vi "Endurance.vi"() -> ()   [LabVIEW 2020]
uses:
  Control/EnduranceIndicator.ctl
  Control/EnduranceBufferControl.ctl
  Control/EnduranceRecordRemove.ctl
  Control/EnduranceCurrentIndicator.ctl
  Control/EnduranceState.ctl
  <vilib>/DAQmx/write.llb/DAQmx Write (Analog DBL 1Chan 1Samp).vi
  <vilib>/DAQmx/read.llb/DAQmx Read (Analog DBL 1Chan 1Samp).vi
  <vilib>/DAQmx/create/channels.llb/DAQmx Create Channel (AO-Voltage-Basic).vi
  <vilib>/DAQmx/create/channels.llb/DAQmx Create Channel (AI-Voltage-Basic).vi
  <vilib>/Utility/file.llb/Read Delimited Spreadsheet (string).vi
  <vilib>/DAQmx/miscellaneous.llb/DAQmx Fill In Error Info.vi
panel:
  out "CurrentIndicator":T1
  out "ElapsedTime":string
  in  "RecordRemove":T2
  in  "BufferControl":T3
  in  "DeviceName":tag
  out "BufferIndicator":T4
  in  "Ready":bool
  in  "Stop":bool
  # "2022 KSAE Formula Endurance  Event"
  # "Record-6:"
  # "Record-7:"
  # "Record-8:"
  # "Record-9:"
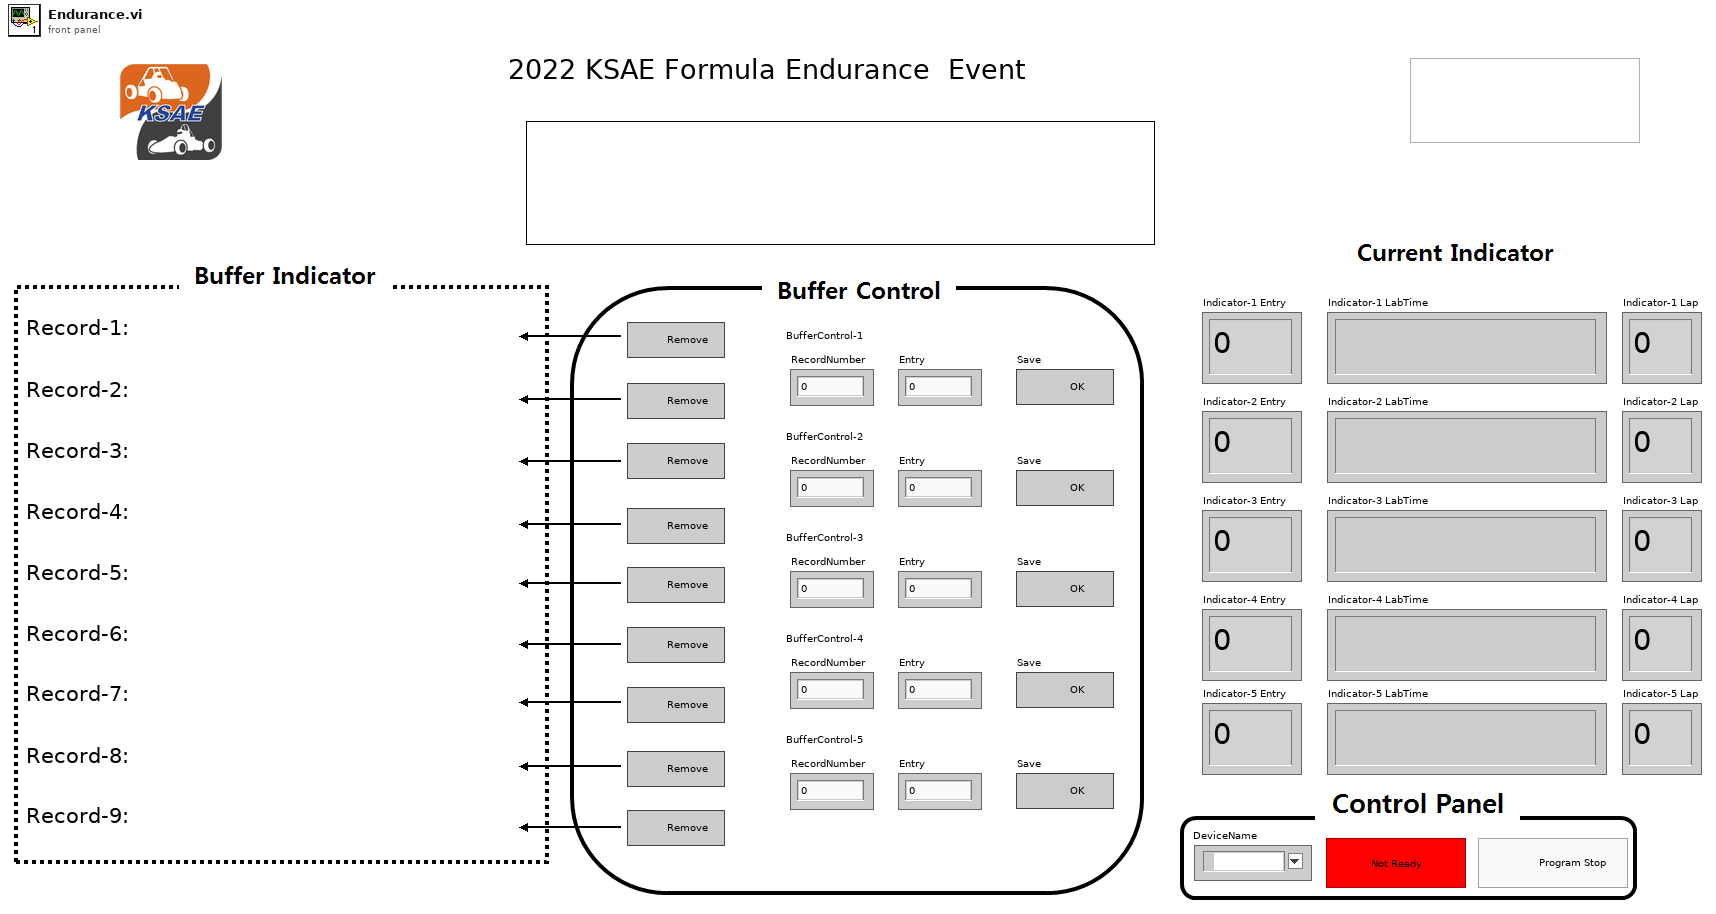
[diagram p1: front panel]
types:
  T1 = typedef "EnduranceCurrentIndicator.ctl" = cluster{"Indicator-1 Entry":u8, "Indicator-1 LabTime":string, "Indicator-1 Lap":u8, "Indicator-2 Entry":u8, "Indicator-2 LabTime":string, "Indicator-2 Lap":u8, "Indicator-3 Entry":u8, "Indicator-3 LabTime":string, "Indicator-3 Lap":u8, "Indicator-4 Entry":u8, "Indicator-4 LabTime":string, "Indicator-4 Lap":u8, "Indicator-5 Entry":u8, "Indicator-5 LabTime":string, "Indicator-5 Lap":u8}
  T2 = typedef "EnduranceRecordRemove.ctl" = cluster{"Record-1 Remove":bool, "Record-2 Remove":bool, "Record-3 Remove":bool, "Record-4 Remove":bool, "Record-5 Remove":bool, "Record-6 Remove":bool, "Record-7 Remove":bool, "Record-8 Remove":bool, "Record-9 Remove":bool}
  T3 = typedef "EnduranceBufferControl.ctl" = cluster{"BufferControl-1":cluster{"RecordNumber":u8, "Entry":u8, "Save":bool}, "BufferControl-2":cluster{"RecordNumber":u8, "Entry":u8, "Save":bool}, "BufferControl-3":cluster{"RecordNumber":u8, "Entry":u8, "Save":bool}, "BufferControl-4":cluster{"RecordNumber":u8, "Entry":u8, "Save ":bool}, "BufferControl-5":cluster{"RecordNumber":u8, "Entry":u8, "Save":bool}}
  T4 = typedef "EnduranceIndicator.ctl" = cluster{"Record-1":string, "Record-2":string, "Record-3":string, "Record-4":string, "Record-5":string, "Record-6":string, "Record-7":string, "Record-8":string, "Record-9":string}
  T5 = typedef "EnduranceState.ctl" = enum16{"Initial", "Ready", "Running", "LoggingData", "ProgramStop"}
  T6 = cluster{"BufferIndicator":T4, "State":T5, "InitialTime":i64, "RecordBuffer":cluster{"RecordBuffer(Time)":i64[], "RecordBuffer(Display)":string[]}, "CurrentIndicator":T1, "BufferControl":T3}
  T7 = cluster{"RecordBuffer(Time)":i64[], "RecordBuffer(Display)":string[]}
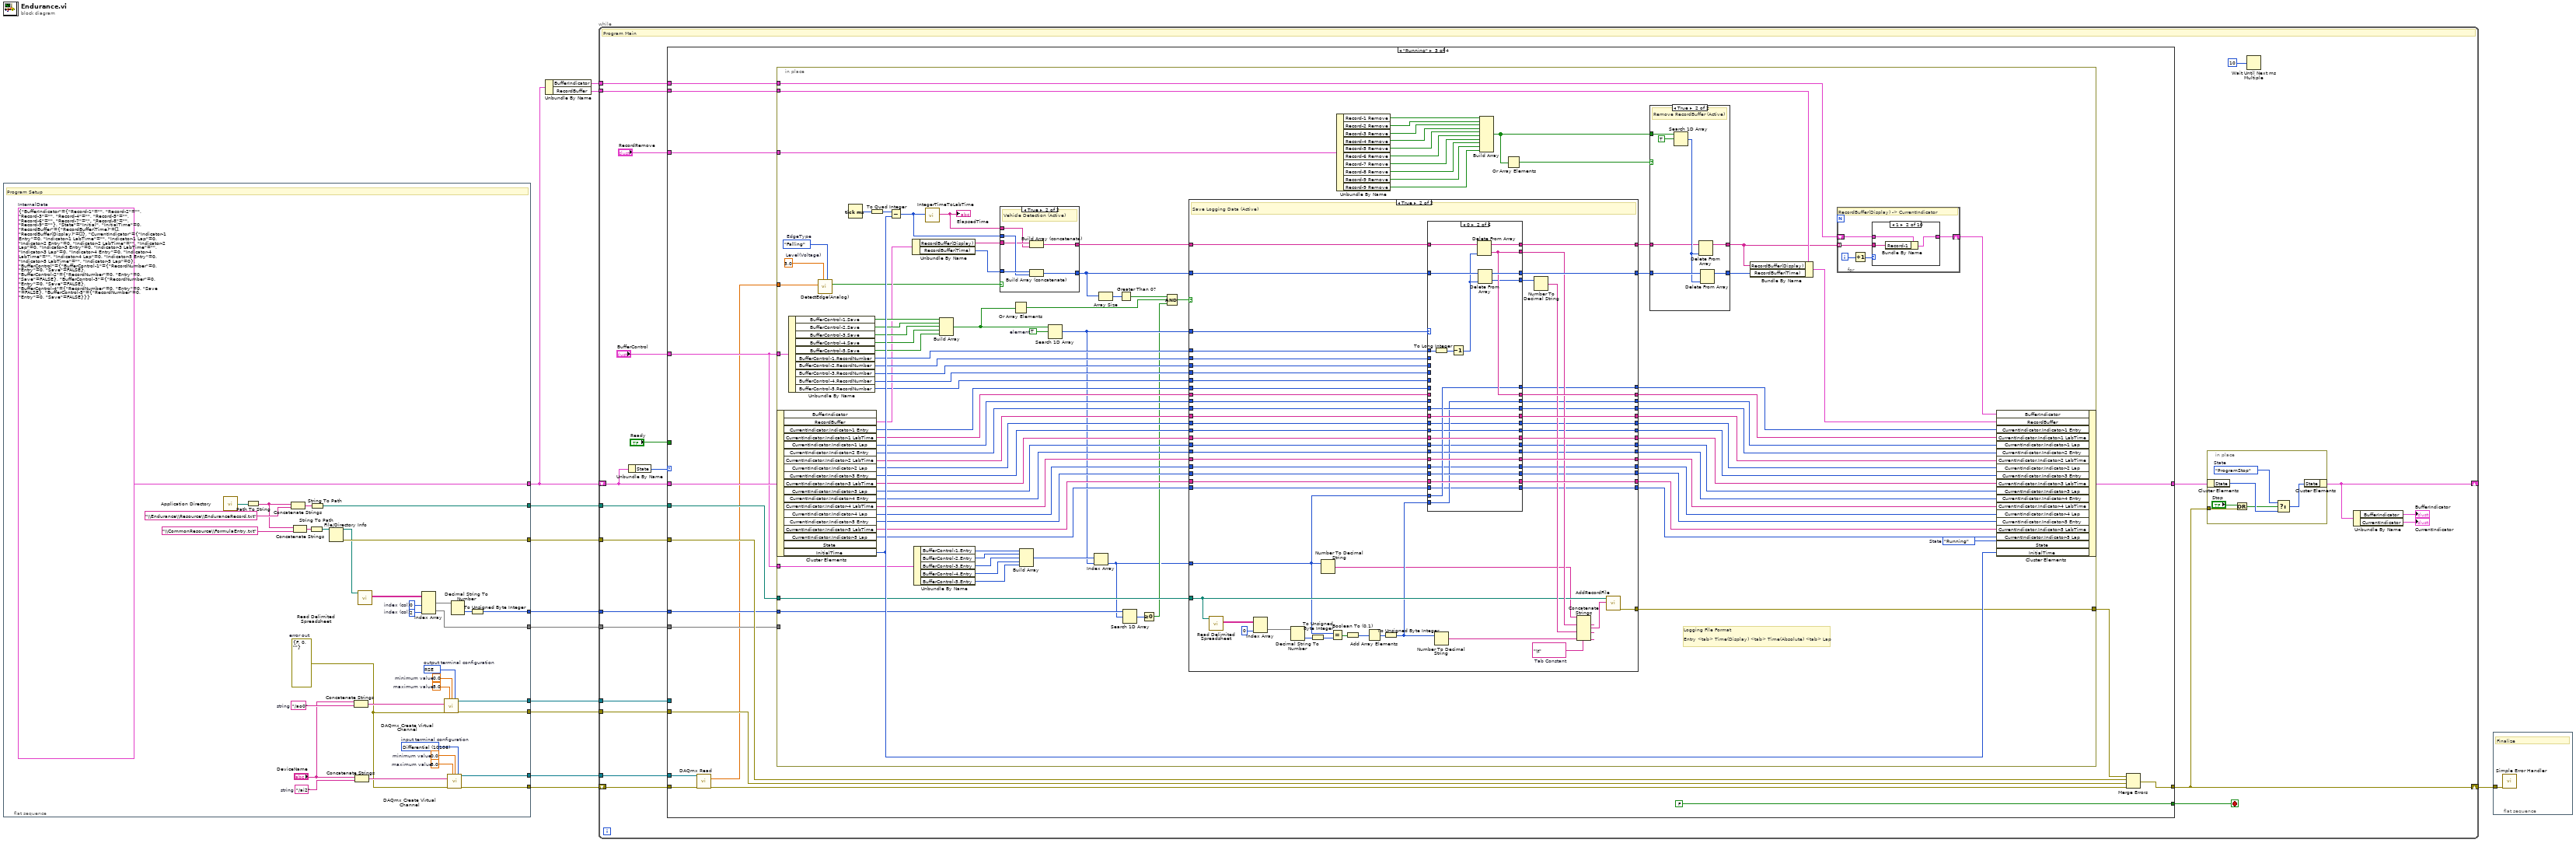
[diagram p0: block diagram]
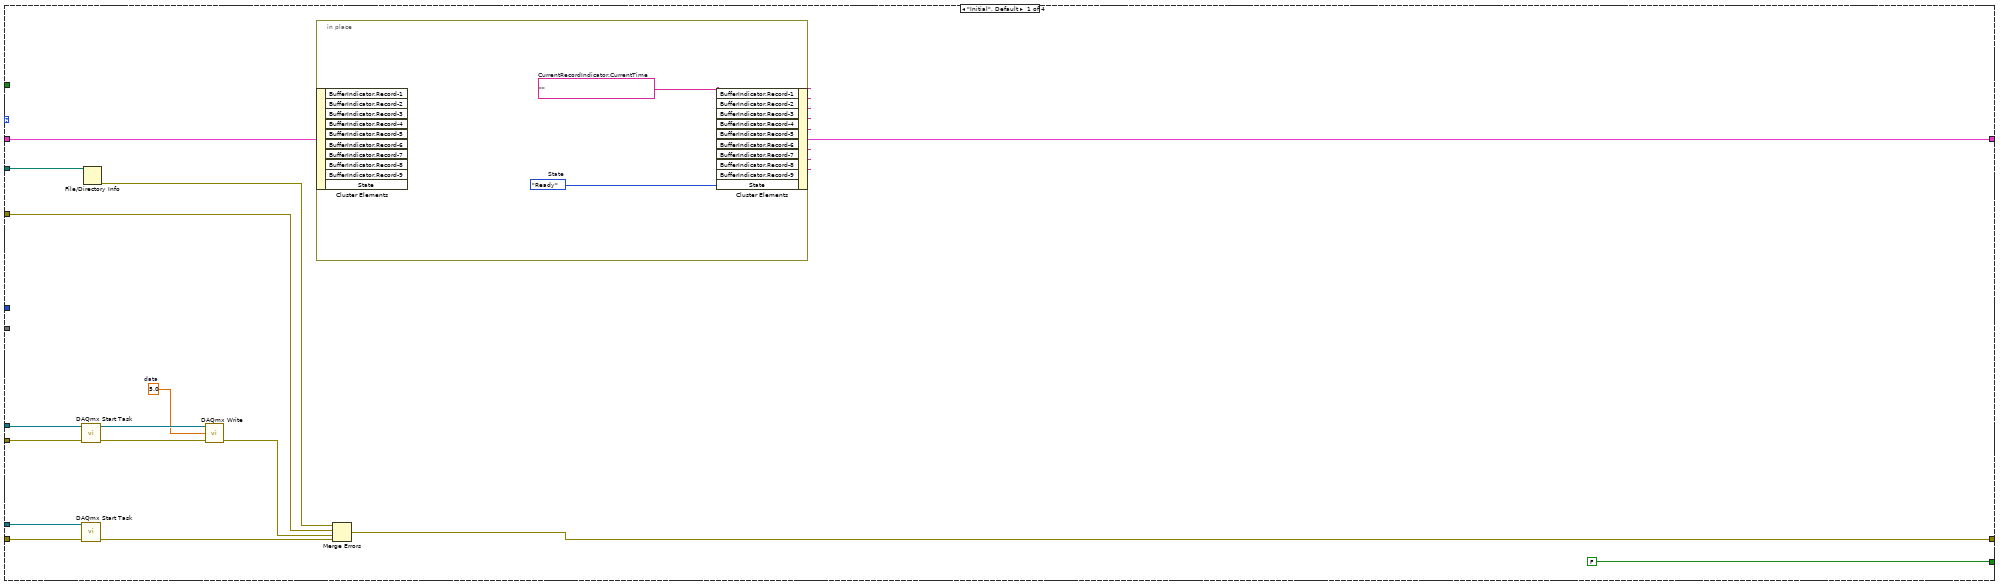
[diagram p2: hidden frame]
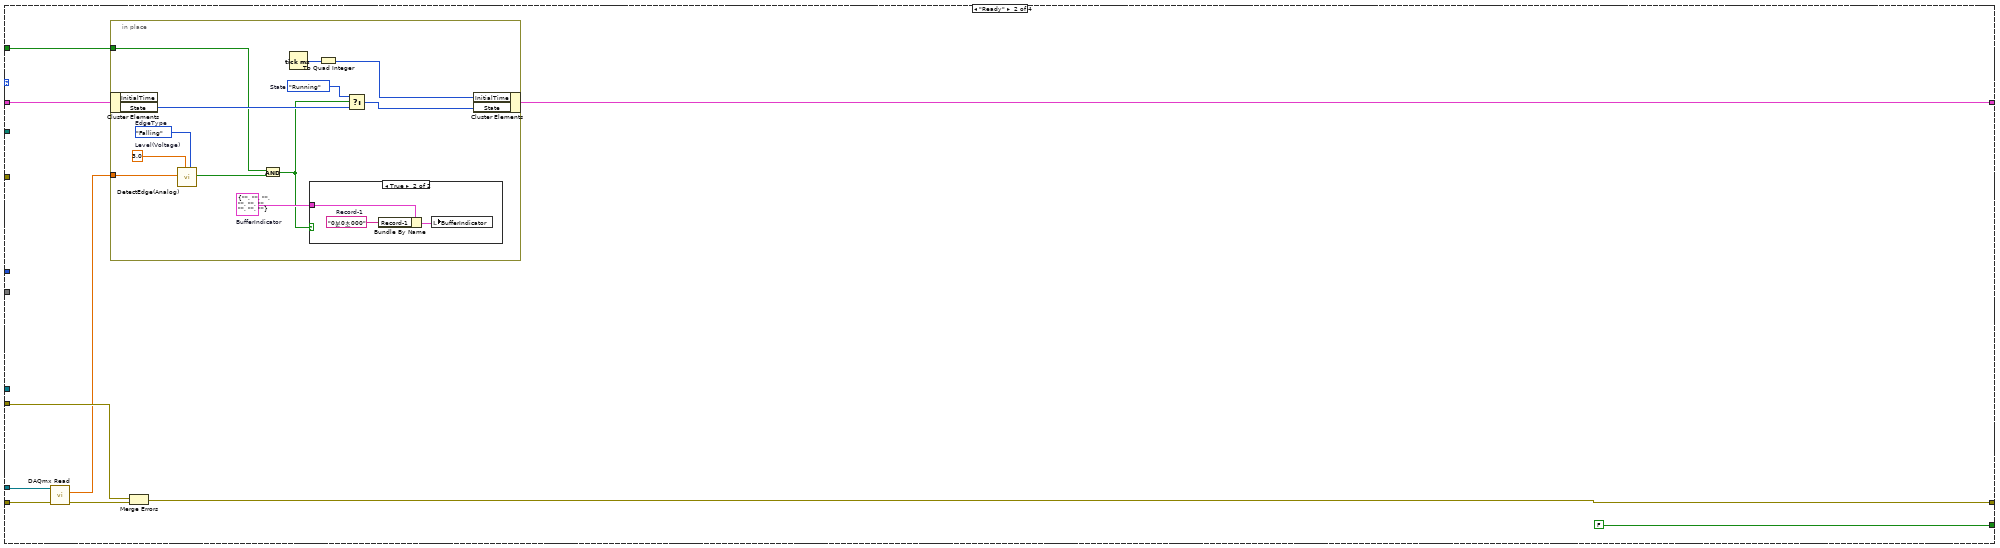
[diagram p3: hidden frame]
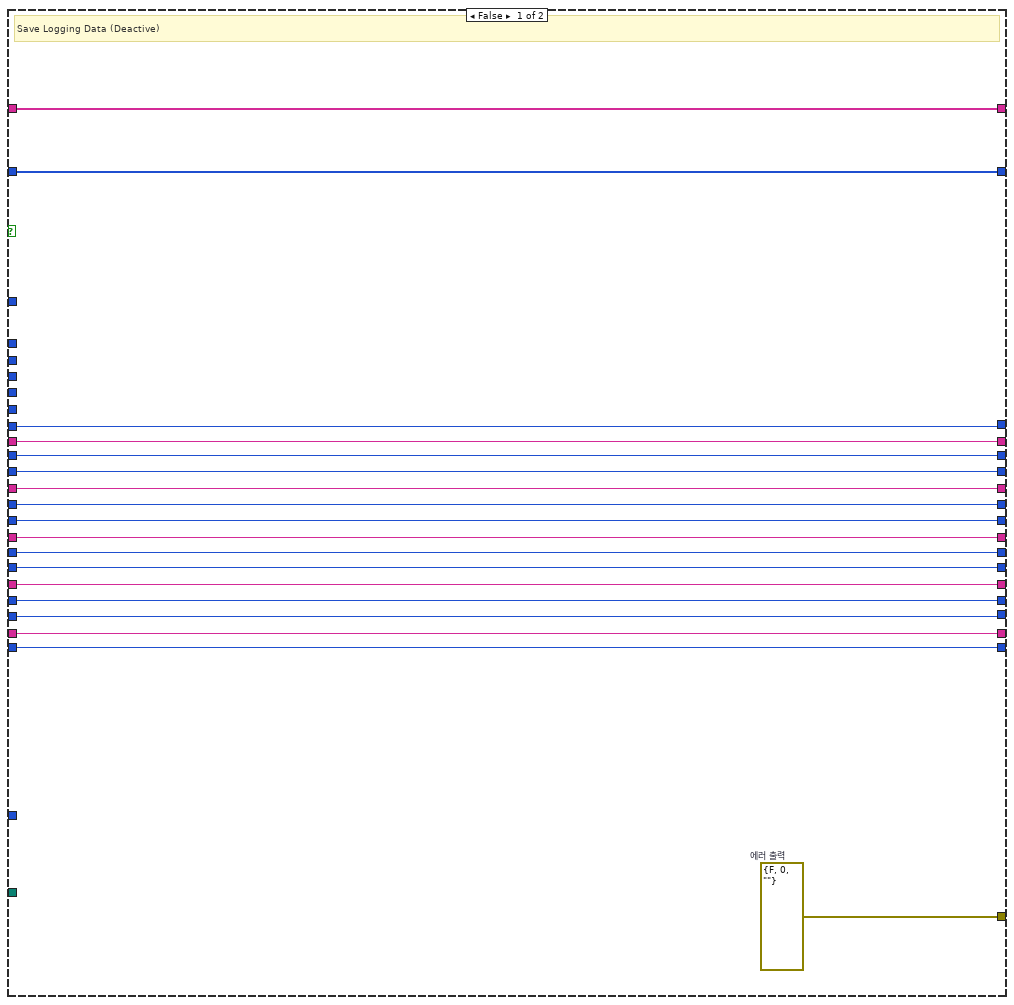
[diagram p6: hidden frame]
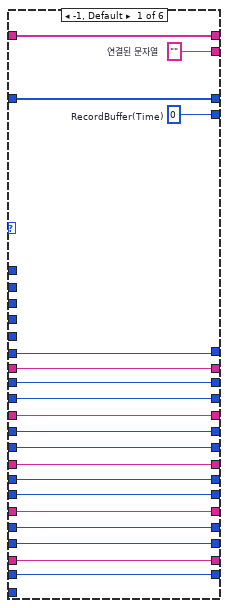
[diagram p7: hidden frame]
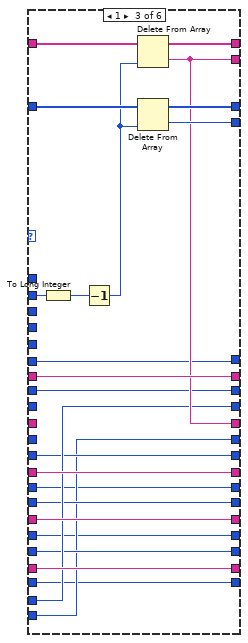
[diagram p8: hidden frame]
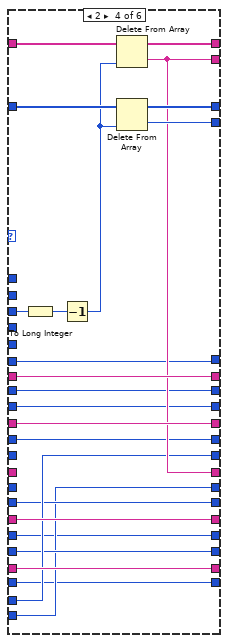
[diagram p9: hidden frame]
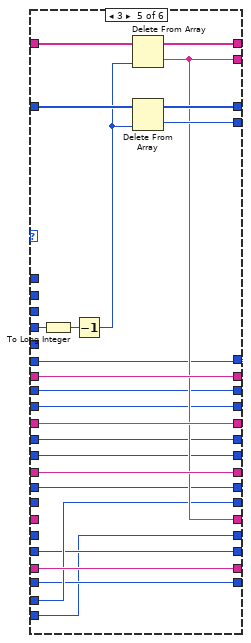
[diagram p10: hidden frame]
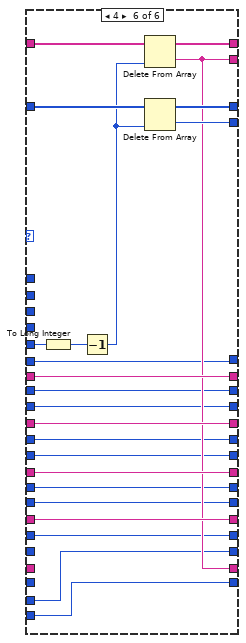
[diagram p11: hidden frame]
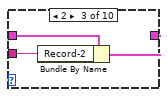
[diagram p14: hidden frame]
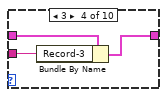
[diagram p15: hidden frame]
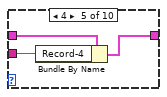
[diagram p16: hidden frame]
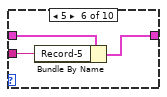
[diagram p17: hidden frame]
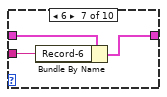
[diagram p18: hidden frame]
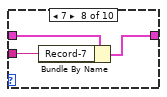
[diagram p19: hidden frame]
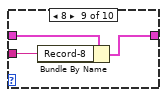
[diagram p20: hidden frame]
diagram:
  n1 = flat-sequence {
    tunnel: [w45] -> w11
    tunnel: [w44] -> w10
    tunnel: [w41] -> w9
    tunnel: [w40] -> w8
    tunnel: [w36] -> w6
    tunnel: [w27] -> w7
    tunnel: [w22] -> w3
    tunnel: [w15] -> w2
    tunnel: [w17] -> w1
    frame #0 {
      w13 = errorcluster {"status"=FALSE, "code"=0, "source"=""}  # error out
      w19 = 2  # index (col)
      w20 = 0  # index (col)
      w36 = T6 {"BufferIndicator"={"Record-1"="", "Record-2"="", "Record-3"="", "Record-4"="", "Record-5"="", "Record-6"="", "Record-7"="", "Record-8"="", "Record-9"=""}, "State"=enum."Initial", "InitialTime"=0, "RecordBuffer"={"RecordBuffer(Time)"=[], "RecordBuffer(Display)"=[]}, "CurrentIndicator"={"Indicator-1 Entry"=0, "Indicator-1 LabTime"="", "Indicator-1 Lap"=0, "Indicator-2 Entry"=0, "Indicator-2 LabTime"="", "Indicator-2 Lap"=0, "Indicator-3 Entry"=0, "Indicator-3 LabTime"="", "Indicator-3 Lap"=0, "Indicator-4 Entry"=0, "Indicator-4 LabTime"="", "Indicator-4 Lap"=0, "Indicator-5 Entry"=0, "Indicator-5 LabTime"="", "Indicator-5 Lap"=0}, "BufferControl"={"BufferControl-1"={"RecordNumber"=0, "Entry"=0, "Save"=FALSE}, "BufferControl-2"={"RecordNumber"=0, "Entry"=0, "Save"=FALSE}, "BufferControl-3"={"RecordNumber"=0, "Entry"=0, "Save"=FALSE}, "BufferControl-4"={"RecordNumber"=0, "Entry"=0, "Save "=FALSE}, "BufferControl-5"={"RecordNumber"=0, "Entry"=0, "Save"=FALSE}}}  # InternalData
      w33 = "/ai2"  # string
      w35 = "/ao0"  # string
      w37 = 10083 items=["Default"=-1, "RSE"=10083, "Differential"=10106, "Pseudodifferential"=12529]  # output terminal configuration
      w38 = 0.0  # minimum value
      w39 = 5.0  # maximum value
      w43 = 5.0  # maximum value
      w42 = 0.0  # minimum value
      w46 = 10106 items=["default"=-1, "RSE"=10083, "NRSE"=10078, "Differential"=10106, "Pseudodifferential"=12529]  # input terminal configuration
      # "Program Setup"
      n2 = call <vilib>:"Application Directory.vi"() -> ("Application Directory"=w30:path)
      n3 = Path To String(path=w30) -> (string=w24:string)
      n4 = Concatenate Strings "Concatenate Strings"(w24, "\\Endurance\\Resource\\EnduranceRecord.txt") -> (w28:string)
      n5 = Concatenate Strings "Concatenate Strings"(w24, "\\CommonResource\\FormulaEntry.txt") -> (w25:string)
      n6 = String To Path(string=w25) -> (path=w23:path)
      n7 = String To Path(string=w28) -> (path=w27:path)
      n8 = File/Directory Info(path=w23) -> (path out=w21:path, error out=w22:errorcluster)  [unwired: 1 in, 5 out]
      n9 = Concatenate Strings "Concatenate Strings"("DeviceName", w35) -> (w32:string)
      n10 = Concatenate Strings "Concatenate Strings"("DeviceName", w33) -> (w31:string)
      n11 = call-poly <vilib>:"Read Delimited Spreadsheet.vi"("file path (dialog if empty)"=w21) -> ("all rows"=w14:string[][])  [unwired: 9 in, 5 out]
      n12 = Index Array "Index Array"(array=w14, index (col) #1=w20, index (col) #2=w19) -> (element #1=w18:string[], element #2=w17:string[])  [unwired: 2 in]
      n13 = call-poly <vilib>:"DAQmx Create Virtual Channel.vi"("maximum value"=w39, "minimum value"=w38, "output terminal configuration"=w37, "physical channels"=w32, "error in"=w13) -> ("task out"=w41:refnum<k21>, "error out"=w40:errorcluster)  [unwired: 9 in]
      n14 = call-poly <vilib>:"DAQmx Create Virtual Channel.vi"("maximum value"=w43, "minimum value"=w42, "input terminal configuration"=w46, "physical channels"=w31, "error in"=w13) -> ("task out"=w44:refnum<k21>, "error out"=w45:errorcluster)  [unwired: 9 in]
      n15 = Decimal String To Number(string=w18) -> (number=w16:i32[])  [unwired: 2 in, 1 out]
      n16 = To Unsigned Byte Integer(number=w16) -> (unsigned 8bit integer=w15:u8[])
    }
  }
  n17 = Unbundle By Name(w6) -> ("BufferIndicator"=w4:T4, "RecordBuffer"=w5:T7)
  n18 = while {
    tunnel: w10 -> [w68]
    shift-right: [w58] -> _
    shift-left: w6 -> [w65]
    shift-right: [w62] -> w12
    shift-left: w11 -> [w67]
    tunnel: w9 -> [w60]
    tunnel: w8 -> [w59]
    tunnel: w7 -> [w54]
    tunnel: w5 -> [w53]
    tunnel: w4 -> [w52]
    tunnel: w3 -> [w50]
    tunnel: w2 -> [w49]
    tunnel: w1 -> [w48]
    stop <- w63 stop-if-true
    # "Program Main"
    n19 = Unbundle By Name(w65) -> ("State"=w66:T5)
    n20 = case shown="\"Running\"" w66 {
      tunnel: w68 -> [w77 w96 w129 w495]
      tunnel: w67 -> [w78 w95 w128 w498]
      tunnel: w65 -> [w84 w94 w125 w497]
      tunnel: [w83 w93 w126 w496] -> w64
      tunnel: [FALSE FALSE FALSE TRUE] -> w63
      tunnel: [w81 w89 w124 w490] -> w62
      tunnel: "Ready" -> [_ w90 _ _]
      tunnel: w60 -> [w74 _ _ w492]
      tunnel: w59 -> [w75 w88 w123 w491]
      tunnel: "BufferControl" -> [_ _ w118 _]
      tunnel: "RecordRemove" -> [_ _ w121 _]
      tunnel: w54 -> [w70 _ w120 _]
      tunnel: w53 -> [_ _ w117 _]
      tunnel: w52 -> [_ _ w116 _]
      tunnel: w50 -> [w69 _ w115 w488]
      tunnel: w49 -> [_ _ w114 _]
      tunnel: w48 -> [_ _ w113 _]
      frame "Initial", Default {
        w72 = 5.0  # data
        n21 = call <vilib>:"DAQmx Start Task.vi"("task/channels in"=w74, "error in"=w75) -> ("task out"=w80:refnum<k21>, "error out"=w79:errorcluster)  [unwired: 12 in]
        n22 = call <vilib>:"DAQmx Start Task.vi"("task/channels in"=w77, "error in"=w78) -> ("error out"=w76:errorcluster)  [unwired: 12 in, 1 out]
        n23 = File/Directory Info(path=w70) -> (error out=w71:errorcluster)  [unwired: 1 in, 6 out]
        n24 = call-poly <vilib>:"DAQmx Write.vi"("task/channels in"=w80, "data"=w72, "error in"=w79) -> ("error out"=w73:errorcluster)  [unwired: 10 in, 2 out]
        n25 = in-place {
          w85 = EnduranceState."Ready"  # State
          w86 = ""  # CurrentRecordIndicator.CurrentTime
          n26 = in-place-cluster #1(w84) -> ()  [unwired: 10 out]
          n27 = in-place-cluster #1("BufferIndicator.Record-1"=w86, "BufferIndicator.Record-2"=w86, "BufferIndicator.Record-3"=w86, "BufferIndicator.Record-4"=w86, "BufferIndicator.Record-5"=w86, "BufferIndicator.Record-6"=w86, "BufferIndicator.Record-7"=w86, "BufferIndicator.Record-8"=w86, "BufferIndicator.Record-9"=w86, "State"=w85) -> (w83:T6)
        }
        n28 = Merge Errors "Merge Errors"(w71, w69, w73, w76) -> (w81:errorcluster)
      }
      frame "Ready" {
        n29 = call-poly <vilib>:"DAQmx Read.vi"("task/channels in"=w96, "error in"=w95) -> ("data"=w87:dbl, "error out"=w91:errorcluster)  [unwired: 11 in, 1 out]
        n30 = in-place {
          in-place-border: w87 -> [w105]
          in-place-border: w90 -> [w103]
          w98 = enum16{"Rising", "Falling"}."Falling"  # EdgeType
          w100 = T4 {"Record-1"="", "Record-2"="", "Record-3"="", "Record-4"="", "Record-5"="", "Record-6"="", "Record-7"="", "Record-8"="", "Record-9"=""}  # BufferIndicator
          w102 = EnduranceState."Running"  # State
          w104 = 3.0  # Level(Voltage)
          n31 = in-place-cluster #2(w94) -> ("State"=w108:T5)  [unwired: 1 out]
          n32 = call "DetectEdge(Analog).vi"("EdgeType"=w98, "Level(Voltage)"=w104, "Voltage"=w105) -> ("DetectedEdge"=w106:bool)  [unwired: 8 in]
          n33 = And(x=w103, y=w106) -> (x .and. y?=w99:bool)
          n34 = Tick Count (ms)() -> (millisecond timer value=w101:u32)
          n35 = case shown="True" w99 {
            tunnel: w100 -> [_ w111]
            frame False {
            }
            frame True {
              w109 = "0분0초000"  # Record-1
              n36 = Bundle By Name(cluster=w111, "Record-1"=w109) -> (w110:T4)
              n37 = local write "BufferIndicator"(w110) -> ()
            }
          }
          n38 = To Quad Integer(1:w101) -> (0:w97:i64)
          n39 = Select(t=w102, s=w99, f=w108) -> (s? t:f=w107:T5)
          n40 = in-place-cluster #2("InitialTime"=w97, "State"=w107) -> (w93:T6)
        }
        n41 = Merge Errors "Merge Errors"(w88, w91) -> (w89:errorcluster)
      }
      frame "Running" {
        n42 = call-poly <vilib>:"DAQmx Read.vi"("task/channels in"=w129, "error in"=w128) -> ("data"=w112:dbl, "error out"=w122:errorcluster)  [unwired: 11 in, 1 out]
        n43 = in-place {
          in-place-border: w112 -> [w224]
          in-place-border: w118 -> [w183]
          in-place-border: w121 -> [w214]
          in-place-border: w120 -> [w185]
          in-place-border: [w184] -> w119
          in-place-border: w118 -> [w182]
          in-place-border: w117 -> [w172]
          in-place-border: w116 -> [w170]
          in-place-border: w114 -> [w135]
          in-place-border: w113 -> [_]
          w130 = enum16{"Rising", "Falling"}."Falling"  # EdgeType
          w144 = TRUE  # element
          w169 = EnduranceState."Running"  # State
          w226 = 3.0  # Level(Voltage)
          # "Logging File Format\n\nEntry <tab> Time(Display) <tab> Time(Absolute) <tab> Lap"
          n44 = in-place-cluster #3(w125) -> ("RecordBuffer"=w178:T7, "CurrentIndicator.Indicator-1 Entry"=w167:u8, "CurrentIndicator.Indicator-1 LabTime"=w195:string, "CurrentIndicator.Indicator-1 Lap"=w154:u8, "CurrentIndicator.Indicator-2 Entry"=w165:u8, "CurrentIndicator.Indicator-2 LabTime"=w194:string, "CurrentIndicator.Indicator-2 Lap"=w152:u8, "CurrentIndicator.Indicator-3 Entry"=w163:u8, "CurrentIndicator.Indicator-3 LabTime"=w193:string, "CurrentIndicator.Indicator-3 Lap"=w150:u8, "CurrentIndicator.Indicator-4 Entry"=w161:u8, "CurrentIndicator.Indicator-4 LabTime"=w192:string, "CurrentIndicator.Indicator-4 Lap"=w148:u8, "CurrentIndicator.Indicator-5 Entry"=w159:u8, "CurrentIndicator.Indicator-5 LabTime"=w191:string, "CurrentIndicator.Indicator-5 Lap"=w146:u8, "InitialTime"=w225:i64)  [unwired: 2 out]
          n45 = Unbundle By Name(w183) -> ("BufferControl-1.Save"=w201:bool, "BufferControl-2.Save"=w200:bool, "BufferControl-3.Save"=w199:bool, "BufferControl-4.Save"=w198:bool, "BufferControl-5.Save"=w197:bool, "BufferControl-1.RecordNumber"=w218:u8, "BufferControl-2.RecordNumber"=w217:u8, "BufferControl-3.RecordNumber"=w216:u8, "BufferControl-4.RecordNumber"=w215:u8, "BufferControl-5.RecordNumber"=w168:u8)
          n46 = call "DetectEdge(Analog).vi"("EdgeType"=w130, "Level(Voltage)"=w226, "Voltage"=w224) -> ("DetectedEdge"=w131:bool)  [unwired: 8 in]
          n47 = Tick Count (ms)() -> (millisecond timer value=w223:u32)
          n48 = To Quad Integer(1:w223) -> (0:w222:i64)
          n49 = Subtract(x=w222, y=w225) -> (x-y=w221:i64)
          n50 = Unbundle By Name(w178) -> ("RecordBuffer(Display)"=w176:string[], "RecordBuffer(Time)"=w177:i64[])
          n51 = Unbundle By Name(w182) -> ("BufferControl-1.Entry"=w142:u8, "BufferControl-2.Entry"=w141:u8, "BufferControl-3.Entry"=w140:u8, "BufferControl-4.Entry"=w139:u8, "BufferControl-5.Entry"=w138:u8)
          n52 = call "IntegerTimeToLabTime.vi"("inputTime(msec)"=w221) -> ("outputTime(mm-ss-sss)"=w175:string)  [unwired: 10 in]
          "ElapsedTime" <- w175
          n53 = Build Array "Build Array"(w201, w200, w199, w198, w197) -> (w143:bool[])
          n54 = case shown="True" w131 {
            tunnel: w177 -> [w228 w234]
            tunnel: w221 -> [_ w232]
            tunnel: [w228 w233] -> w181
            tunnel: w176 -> [w227 w231]
            tunnel: w175 -> [_ w230]
            tunnel: [w227 w229] -> w174
            frame False {
              # "Vehicle Detection (Deactive)"
            }
            frame True {
              # "Vehicle Detection (Active)"
              n55 = Build Array (concatenate) "Build Array"(w231, w230) -> (w229:string[])
              n56 = Build Array (concatenate) "Build Array"(w234, w232) -> (w233:i64[])
            }
          }
          n57 = Or Array Elements(Boolean array=w143) -> (logical OR=w180:bool)
          n58 = Build Array "Build Array"(w142, w141, w140, w139, w138) -> (w137:u8[])
          n59 = Search 1D Array(1D array=w143, element=w144) -> (index of element=w136:i32)  [unwired: 1 in]
          n60 = Index Array "Index Array"(array=w137, index=w136) -> (element=w133:u8)
          n61 = Array Size(array=w181) -> (size(s)=w220:i32)
          n62 = Greater Than 0?(x=w220) -> (x > 0?=w196:bool)
          n63 = Search 1D Array(1D array=w135, element=w133) -> (index of element=w132:i32)  [unwired: 1 in]
          n64 = Greater Or Equal To 0?(x=w132) -> (x >= 0?=w134:bool)
          n65 = Compound Arithmetic op=AND(w196, w180, w134) -> (w219:bool)
          n66 = case shown="True" w219 {
            tunnel: w181 -> [w246 w311]
            tunnel: [w246 w294] -> w179
            tunnel: w218 -> [_ w310]
            tunnel: w217 -> [_ w309]
            tunnel: w216 -> [_ w308]
            tunnel: w215 -> [_ w307]
            tunnel: w168 -> [_ w306]
            tunnel: w195 -> [w252 w305]
            tunnel: w194 -> [w251 w304]
            tunnel: w193 -> [w250 w303]
            tunnel: w192 -> [w249 w302]
            tunnel: w191 -> [w248 w301]
            tunnel: [w252 w300] -> w190
            tunnel: [w251 w299] -> w189
            tunnel: [w250 w298] -> w188
            tunnel: [w249 w297] -> w187
            tunnel: [w248 w296] -> w186
            tunnel: w185 -> [_ w278]
            tunnel: [w247 w295] -> w184
            tunnel: [w245 w292] -> w173
            tunnel: w174 -> [w245 w291]
            tunnel: w167 -> [w244 w288]
            tunnel: [w244 w287] -> w166
            tunnel: w165 -> [w243 w286]
            tunnel: [w243 w285] -> w164
            tunnel: w163 -> [w242 w284]
            tunnel: [w242 w283] -> w162
            tunnel: w161 -> [w241 w281]
            tunnel: [w241 w282] -> w160
            tunnel: w159 -> [w240 w280]
            tunnel: [w240 w279] -> w158
            tunnel: w154 -> [w239 w271]
            tunnel: [w239 w272] -> w153
            tunnel: w152 -> [w238 w268]
            tunnel: [w238 w269] -> w151
            tunnel: w150 -> [w237 w267]
            tunnel: [w237 w266] -> w149
            tunnel: w148 -> [w236 w265]
            tunnel: [w236 w264] -> w147
            tunnel: w146 -> [w235 w263]
            tunnel: [w235 w262] -> w145
            tunnel: w136 -> [_ w256]
            tunnel: w133 -> [_ w254]
            frame False {
              w247 = errorcluster {"status"=FALSE, "code"=0, "source"=""}  # 에러 출력
              # "Save Logging Data (Deactive)"
            }
            frame True {
              w258 = "\t"  # Tab Constant
              # "Save Logging Data (Active)"
              n67 = call-poly <vilib>:"Read Delimited Spreadsheet.vi"("file path (dialog if empty)"=w278) -> ("all rows"=w253:string[][])  [unwired: 9 in, 5 out]
              n68 = Index Array "Index Array"(array=w253, index (col)=0) -> (element=w276:string[])  [unwired: 1 in]
              n69 = Decimal String To Number(string=w276) -> (number=w275:i32[])  [unwired: 2 in, 1 out]
              n70 = To Unsigned Byte Integer(number=w275) -> (unsigned 8bit integer=w255:u8[])
              n71 = Number To Decimal String(number=w254) -> (decimal integer string=w261:string)  [unwired: 1 in]
              n72 = Equal?(x=w254, y=w255) -> (x = y?=w274:bool[])
              n73 = Boolean To (0,1)(Boolean=w274) -> (0, 1=w273:i16[])
              n74 = Add Array Elements(numeric array=w273) -> (sum=w260:i16)
              n75 = To Unsigned Byte Integer(number=w260) -> (unsigned 8bit integer=w270:u8)
              n76 = case shown="0" w256 {
                tunnel: [w330 w352 w375 w398 w421 w444] -> w294
                tunnel: w311 -> [w330 w353 w376 w399 w422 w445]
                tunnel: w310 -> [_ w351 _ _ _ _]
                tunnel: w309 -> [_ _ w374 _ _ _]
                tunnel: w308 -> [_ _ _ w397 _ _]
                tunnel: w307 -> [_ _ _ _ w420 _]
                tunnel: w306 -> [_ _ _ _ _ w443]
                tunnel: w305 -> [w329 _ w373 w394 w417 w440]
                tunnel: w304 -> [w328 w349 _ w395 w416 w439]
                tunnel: w303 -> [w327 w348 w371 _ w418 w438]
                tunnel: w302 -> [w326 w347 w370 w393 _ w441]
                tunnel: w301 -> [w325 w346 w369 w392 w415 _]
                tunnel: [w329 w342 w373 w394 w417 w440] -> w300
                tunnel: [w328 w349 w364 w395 w416 w439] -> w299
                tunnel: [w327 w348 w371 w387 w418 w438] -> w298
                tunnel: [w326 w347 w370 w393 w410 w441] -> w297
                tunnel: [w325 w346 w369 w392 w415 w433] -> w296
                tunnel: [w322 w342 w364 w387 w410 w433] -> w293
                tunnel: [w324 w344 w366 w389 w413 w435] -> w292
                tunnel: w291 -> [w324 w345 w367 w390 w412 w436]
                tunnel: [w323 w341 w365 w388 w411 w434] -> w290
                tunnel: [w321 w340 w363 w385 w409 w428] -> w287
                tunnel: w288 -> [w321 _ w363 w385 w409 w428]
                tunnel: w286 -> [w320 w339 _ w384 w407 w432]
                tunnel: [w320 w339 w362 w384 w407 w432] -> w285
                tunnel: [w319 w338 w361 w386 w405 w431] -> w283
                tunnel: w284 -> [w319 w338 w361 _ w405 w431]
                tunnel: [w318 w337 w360 w383 w408 w430] -> w282
                tunnel: w281 -> [w318 w337 w360 w383 _ w430]
                tunnel: w280 -> [w317 w336 w359 w382 w406 _]
                tunnel: [w317 w336 w359 w382 w406 w429] -> w279
                tunnel: w254 -> [_ w340 w362 w386 w408 w429]
                tunnel: [w316 w335 w358 w381 w404 w427] -> w272
                tunnel: w271 -> [w316 _ w358 w381 w404 w427]
                tunnel: w270 -> [_ w335 w357 w379 w400 w424]
                tunnel: [w315 w334 w357 w380 w403 w426] -> w269
                tunnel: w268 -> [w315 w334 _ w380 w403 w426]
                tunnel: w267 -> [w314 w333 w356 _ w402 w425]
                tunnel: [w314 w333 w356 w379 w402 w425] -> w266
                tunnel: w265 -> [w313 w331 w355 w377 _ w423]
                tunnel: [w313 w331 w355 w377 w400 w423] -> w264
                tunnel: w263 -> [w312 w332 w354 w378 w401 _]
                tunnel: [w312 w332 w354 w378 w401 w424] -> w262
                frame -1, Default {
                  w322 = ""  # 연결된 문자열
                  w323 = i64 0  # RecordBuffer(Time)
                }
                frame 0 {
                  n77 = To Long Integer(number=w351) -> (32bit integer=w350:i32)
                  n78 = Decrement(x=w350) -> (x-1=w343:i32)
                  n79 = Delete From Array "Delete From Array"(array=w345, index=w343) -> (deleted portion=w342:string, array with subset deleted=w344:string[])  [unwired: 1 in]
                  n80 = Delete From Array "Delete From Array"(array=w353, index=w343) -> (deleted portion=w341:i64, array with subset deleted=w352:i64[])  [unwired: 1 in]
                }
                frame 1 {
                  n81 = To Long Integer(number=w374) -> (32bit integer=w372:i32)
                  n82 = Decrement(x=w372) -> (x-1=w368:i32)
                  n83 = Delete From Array "Delete From Array"(array=w367, index=w368) -> (deleted portion=w364:string, array with subset deleted=w366:string[])  [unwired: 1 in]
                  n84 = Delete From Array "Delete From Array"(array=w376, index=w368) -> (deleted portion=w365:i64, array with subset deleted=w375:i64[])  [unwired: 1 in]
                }
                frame 2 {
                  n85 = To Long Integer(number=w397) -> (32bit integer=w396:i32)
                  n86 = Decrement(x=w396) -> (x-1=w391:i32)
                  n87 = Delete From Array "Delete From Array"(array=w390, index=w391) -> (deleted portion=w387:string, array with subset deleted=w389:string[])  [unwired: 1 in]
                  n88 = Delete From Array "Delete From Array"(array=w399, index=w391) -> (deleted portion=w388:i64, array with subset deleted=w398:i64[])  [unwired: 1 in]
                }
                frame 3 {
                  n89 = To Long Integer(number=w420) -> (32bit integer=w419:i32)
                  n90 = Decrement(x=w419) -> (x-1=w414:i32)
                  n91 = Delete From Array "Delete From Array"(array=w412, index=w414) -> (deleted portion=w410:string, array with subset deleted=w413:string[])  [unwired: 1 in]
                  n92 = Delete From Array "Delete From Array"(array=w422, index=w414) -> (deleted portion=w411:i64, array with subset deleted=w421:i64[])  [unwired: 1 in]
                }
                frame 4 {
                  n93 = To Long Integer(number=w443) -> (32bit integer=w442:i32)
                  n94 = Decrement(x=w442) -> (x-1=w437:i32)
                  n95 = Delete From Array "Delete From Array"(array=w436, index=w437) -> (deleted portion=w433:string, array with subset deleted=w435:string[])  [unwired: 1 in]
                  n96 = Delete From Array "Delete From Array"(array=w445, index=w437) -> (deleted portion=w434:i64, array with subset deleted=w444:i64[])  [unwired: 1 in]
                }
              }
              n97 = Number To Decimal String(number=w270) -> (decimal integer string=w257:string)  [unwired: 1 in]
              n98 = Number To Decimal String(number=w290) -> (decimal integer string=w289:string)  [unwired: 1 in]
              n99 = Concatenate Strings "Concatenate Strings"(w261, w258, w293, w258, w289, w258, w257) -> (w259:string)
              n100 = call "AddRecordFile.vi"("LabTime"=w259, "파일 경로(대화 상자 사용)"=w278) -> ("에러 출력"=w295:errorcluster)  [unwired: 8 in, 1 out]
            }
          }
          n101 = Unbundle By Name(w214) -> ("Record-1 Remove"=w213:bool, "Record-2 Remove"=w212:bool, "Record-3 Remove"=w211:bool, "Record-4 Remove"=w210:bool, "Record-5 Remove"=w209:bool, "Record-6 Remove"=w208:bool, "Record-7 Remove"=w207:bool, "Record-8 Remove"=w206:bool, "Record-9 Remove"=w205:bool, "Record-9 Remove"=w204:bool)
          n102 = Build Array "Build Array"(w213, w212, w211, w210, w209, w208, w207, w206, w205, w204) -> (w202:bool[])
          n103 = Or Array Elements(Boolean array=w202) -> (logical OR=w203:bool)
          n104 = case shown="True" w203 {
            tunnel: w179 -> [w447 w454]
            tunnel: [w447 w451] -> w171
            tunnel: w202 -> [_ w453]
            tunnel: [w446 w449] -> w155
            tunnel: w173 -> [w446 w448]
            frame False {
              # "Remove RecordBuffer (Deactive)"
            }
            frame True {
              # "Remove RecordBuffer (Active)"
              n105 = Search 1D Array(1D array=w453, element=TRUE) -> (index of element=w450:i32)  [unwired: 1 in]
              n106 = Delete From Array "Delete From Array"(array=w448, index=w450) -> (array with subset deleted=w449:string[])  [unwired: 1 in, 1 out]
              n107 = Delete From Array "Delete From Array"(array=w454, index=w450) -> (array with subset deleted=w451:i64[])  [unwired: 1 in, 1 out]
            }
          }
          n108 = Bundle By Name(cluster=w172, "RecordBuffer(Display)"=w155, "RecordBuffer(Time)"=w171) -> (w157:T7)
          n109 = for {
            tunnel: w155 -> [w457] mode=indexing
            shift-right: [w455] -> w156
            shift-left: w170 -> [w456]
            i -> [w459]
            # "RecordBuffer(Display) -> CurrentIndicator"
            n110 = Increment(x=w459) -> (x+1=w458:i32)
            n111 = case shown="1" w458 {
              tunnel: [w460 w463 w466 w469 w472 w475 w478 w481 w484 w487] -> w455
              tunnel: w457 -> [_ w462 w465 w468 w471 w474 w477 w480 w483 w486]
              tunnel: w456 -> [w460 w461 w464 w467 w470 w473 w476 w479 w482 w485]
              frame 0, Default {
              }
              frame 1 {
                n112 = Bundle By Name(cluster=w461, "Record-1"=w462) -> (w463:T4)
              }
              frame 2 {
                n113 = Bundle By Name(cluster=w464, "Record-2"=w465) -> (w466:T4)
              }
              frame 3 {
                n114 = Bundle By Name(cluster=w467, "Record-3"=w468) -> (w469:T4)
              }
              frame 4 {
                n115 = Bundle By Name(cluster=w470, "Record-4"=w471) -> (w472:T4)
              }
              frame 5 {
                n116 = Bundle By Name(cluster=w473, "Record-5"=w474) -> (w475:T4)
              }
              frame 6 {
                n117 = Bundle By Name(cluster=w476, "Record-6"=w477) -> (w478:T4)
              }
              frame 7 {
                n118 = Bundle By Name(cluster=w479, "Record-7"=w480) -> (w481:T4)
              }
              frame 8 {
                n119 = Bundle By Name(cluster=w482, "Record-8"=w483) -> (w484:T4)
              }
              frame 9 {
                n120 = Bundle By Name(cluster=w485, "Record-9"=w486) -> (w487:T4)
              }
            }
          }
          n121 = in-place-cluster #3("BufferIndicator"=w156, "RecordBuffer"=w157, "CurrentIndicator.Indicator-1 Entry"=w166, "CurrentIndicator.Indicator-1 LabTime"=w190, "CurrentIndicator.Indicator-1 Lap"=w153, "CurrentIndicator.Indicator-2 Entry"=w164, "CurrentIndicator.Indicator-2 LabTime"=w189, "CurrentIndicator.Indicator-2 Lap"=w151, "CurrentIndicator.Indicator-3 Entry"=w162, "CurrentIndicator.Indicator-3 LabTime"=w188, "CurrentIndicator.Indicator-3 Lap"=w149, "CurrentIndicator.Indicator-4 Entry"=w160, "CurrentIndicator.Indicator-4 LabTime"=w187, "CurrentIndicator.Indicator-4 Lap"=w147, "CurrentIndicator.Indicator-5 Entry"=w158, "CurrentIndicator.Indicator-5 LabTime"=w186, "CurrentIndicator.Indicator-5 Lap"=w145, "State"=w169, "InitialTime"=w225) -> (w126:T6)
        }
        n122 = Merge Errors "Merge Errors"(w119, w115, w123, w122) -> (w124:errorcluster)
      }
      frame "ProgramStop" {
        n123 = call <vilib>:"DAQmx Clear Task.vi"("task in"=w492, "error in"=w491) -> ("error out"=w489:errorcluster)  [unwired: 13 in]
        n124 = call <vilib>:"DAQmx Clear Task.vi"("task in"=w495, "error in"=w498) -> ("error out"=w494:errorcluster)  [unwired: 13 in]
        n125 = flat-sequence {
          tunnel: w494 -> [w501]
          tunnel: [w501] -> w493
          frame #0 {
            w500 = FALSE  # Ready
            n126 = local write "Ready"(w500) -> ()
          }
        }
        n127 = in-place {
          w502 = EnduranceState."ProgramStop"  # State
          n128 = in-place-cluster #4(w497) -> ()  [unwired: 1 out]
          n129 = in-place-cluster #4("State"=w502) -> (w496:T6)
        }
        n130 = Merge Errors "Merge Errors"(w488, w489, w493) -> (w490:errorcluster)
      }
    }
    n131 = in-place {
      in-place-border: w62 -> [w504]
      w503 = EnduranceState."ProgramStop"  # State
      n132 = in-place-cluster #5(w64) -> ("State"=w507:T5)
      n133 = Or(x="Stop", y=w504) -> (x .or. y?=w505:bool)
      n134 = Select(t=w503, s=w505, f=w507) -> (s? t:f=w506:T5)
      n135 = in-place-cluster #5("State"=w506) -> (w58:T6)
    }
    n136 = Wait Until Next ms Multiple(millisecond multiple=u32 10) -> ()  [unwired: 1 out]
    n137 = Unbundle By Name(w58) -> ("BufferIndicator"=→"BufferIndicator":T4, "CurrentIndicator"=→"CurrentIndicator":T1)
  }
  n138 = flat-sequence {
    tunnel: w12 -> [w509]
    frame #0 {
      # "Finalize"
      n139 = call <vilib>:"Simple Error Handler.vi"("error in (no error)"=w509) -> ()  [unwired: 4 in, 5 out]
    }
  }
